vi "lo lseek.vi"(7 "whence":i32, 8 "error in (no error)":errorcluster, 9 "offset":i32, 10 "fd":i32) -> (0 "error out":errorcluster, 2 "return type":i32)   [LabVIEW 2019, in "libpqlv.lvlib"]
uses:
  libpqlv.lvlib
  libpq.dll
panel:
  in  "conn":u32
  out "conn_out":u32
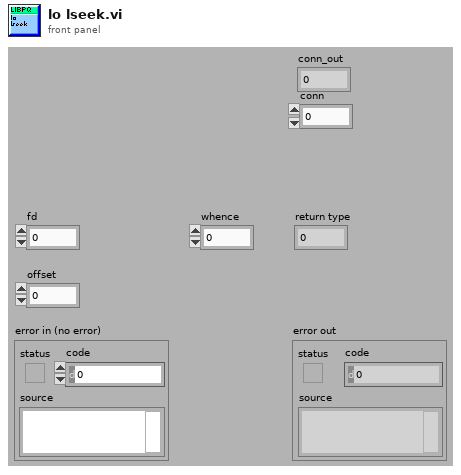
[diagram p1: front panel]
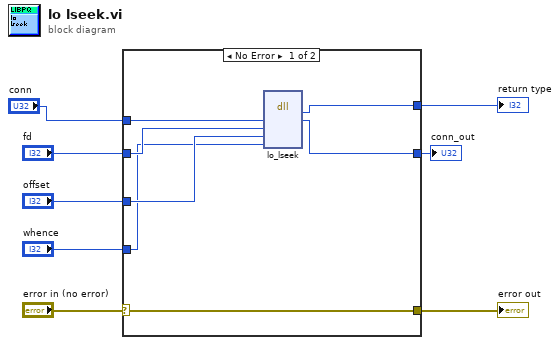
[diagram p0: block diagram]
diagram:
  n1 = case shown="No Error" "error in (no error)" {
    selector: "error in (no error)" -> [w15 w17]
    tunnel: [w15 w17] -> w7
    tunnel: [w14 _] -> w6
    tunnel: [w13 w16] -> w2
    tunnel: "fd" -> [w12 _]
    tunnel: "offset" -> [w11 _]
    tunnel: "whence" -> [w10 _]
    tunnel: "conn" -> [w9 w16]
    frame No Error {
      n2 = dll-call lib="libpq.*" fn="lo_lseek"("conn"=w9, "fd"=w12, "offset"=w11, "whence"=w10) -> ("lo_lseek"=w14:i32, "conn"=w13:u32)  [unwired: 6 in, 2 out]
    }
    frame Error {
    }
  }
  "return type" <- w6
  "error out" <- w7
  "conn_out" <- w2
